vi "Create Data Queues.vi"(8 "error in (no error)":errorcluster) -> (0 "error out":errorcluster, 3 "DataQueuesAndNotifier Out":T1)   [LabVIEW 2019]
uses:
  Support/Data Cluster.ctl
  controls/ImageInfo.ctl
  <vilib>/vision/Image Controls.llb/IMAQ Image.ctl
  Acquisition/DataQueuesAndNotifier.ctl
panel:
  in  "Data Cluster":T2
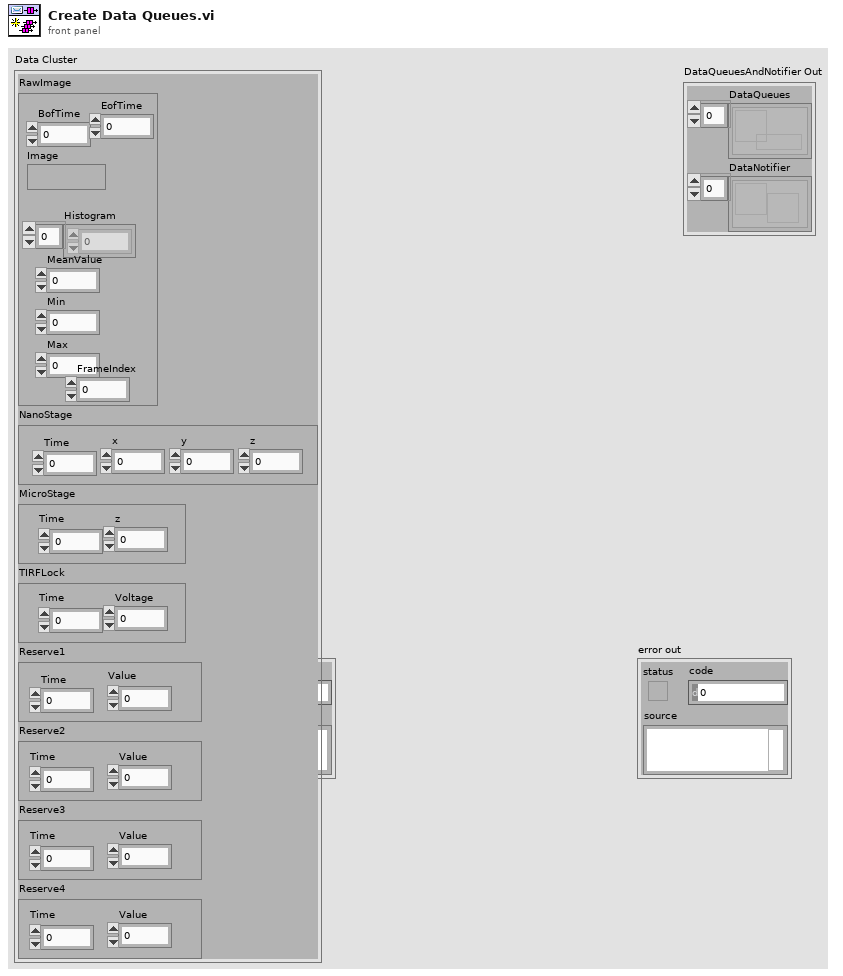
[diagram p1: front panel]
types:
  T1 = typedef "DataQueuesAndNotifier.ctl" = cluster{"DataQueues":refnum<queue>[], "DataNotifier":refnum<notifier>[]}
  T2 = typedef "Data Cluster.ctl" = cluster{"RawImage":T3, "NanoStage":cluster{"Time":dbl, "x":dbl, "y":dbl, "z":dbl}, "MicroStage":cluster{"Time":dbl, "z":dbl}, "TIRFLock":cluster{"Time":dbl, "Voltage":dbl}, "Reserve1":cluster{"Value":dbl, "Time":dbl}, "Reserve2":cluster{"Value":dbl, "Time":dbl}, "Reserve3":cluster{"Value":dbl, "Time":dbl}, "Reserve4":cluster{"Value":dbl, "Time":dbl}}
  T3 = typedef "ImageInfo.ctl" = cluster{"BofTime":dbl, "Image":T4, "Histogram":u32[], "MeanValue":dbl, "Min":u32, "Max":u32, "FrameIndex":dbl, "EofTime":dbl}
  T4 = typedef "IMAQ Image.ctl" = refnum<image>
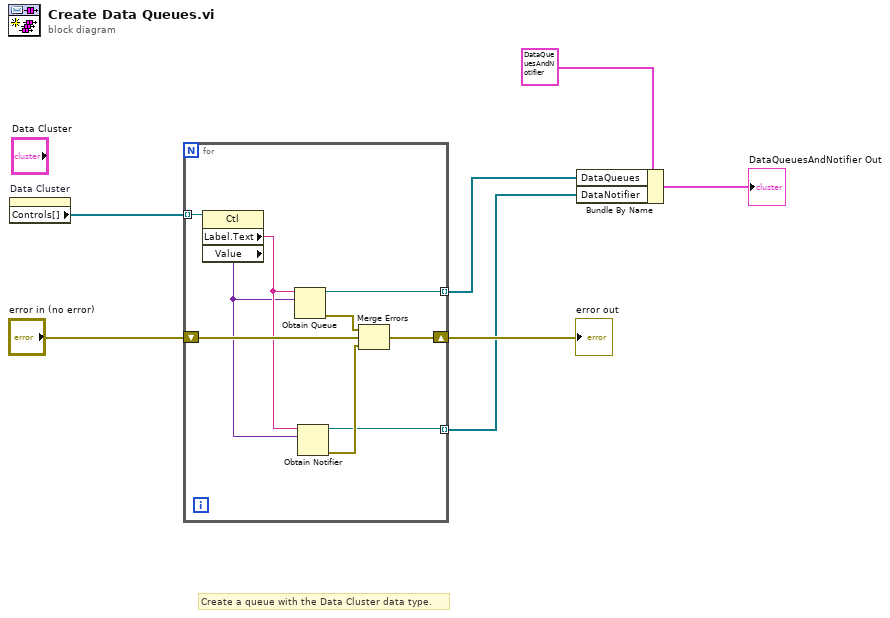
[diagram p0: block diagram]
diagram:
  # "Create a queue with the Data Cluster data type."
  n1 = property on="Data Cluster" class="Clust (strict)"() -> ("Controls[]"=w5:refnum<vi>[])  [unwired: 2 in, 2 out]
  n2 = for {
    shift-right: [w14] -> w6
    shift-left: "error in (no error)" -> [w16]
    tunnel: w5 -> [w13] mode=indexing
    tunnel: [w12] -> w3 mode=indexing
    tunnel: [w8] -> w2 mode=indexing
    n3 = property class="Ctl"(reference=w13) -> ("Label.Text"=w11:string, "Value"=w10:variant)  [unwired: 1 in, 2 out]
    n4 = Obtain Queue(name (unnamed)=w11, element data type=w10) -> (queue out=w12:refnum<queue>, error out=w15:errorcluster)  [unwired: 3 in, 1 out]
    n5 = Obtain Notifier(name (unnamed)=w11, notification data type=w10) -> (notifier out=w8:refnum<notifier>, error out=w9:errorcluster)  [unwired: 2 in, 1 out]
    n6 = Merge Errors(w15, w16, w9) -> (w14:errorcluster)
  }
  "error out" <- w6
  n7 = Bundle By Name(cluster=T1 {"DataQueues"=[refnum, refnum, refnum, refnum, refnum, refnum, refnum, refnum], "DataNotifier"=[refnum, refnum, refnum, refnum, refnum, refnum, refnum, refnum]} ("DataQueuesAndNotifier"), "DataQueues"=w3, "DataNotifier"=w2) -> (→"DataQueuesAndNotifier Out":T1)
